vi "FctioTest.vi"(8 "error in":errorcluster, 9 "Invert Switch":bool, 10 "FPGA Reference In":refnum<k20>, 11 "DAQmx Task Name":refnum<k21>) -> (0 "error out":errorcluster, 2 "Individual Pin Result":bool[](array[boolean]), 3 "Test Pass":bool)   [LabVIEW 2018]
uses:
  Resources_Test/UART/ControlTestSlot.ctl
  <vilib>/DAQmx/read.llb/DAQmx Read (Digital 1D Bool NChan 1Samp 1Line).vi
  <vilib>/DAQmx/miscellaneous.llb/DAQmx Fill In Error Info.vi
panel:
  in  "Enum":T1
  in  "Resp Timeout":i32
  out "data":bool[](array[boolean])
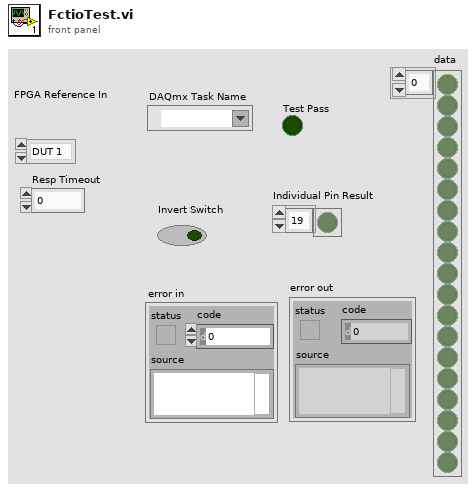
[diagram p1: front panel]
types:
  T1 = typedef "ControlTestSlot.ctl" = enum16{"DUT 1", "DUT 2"}
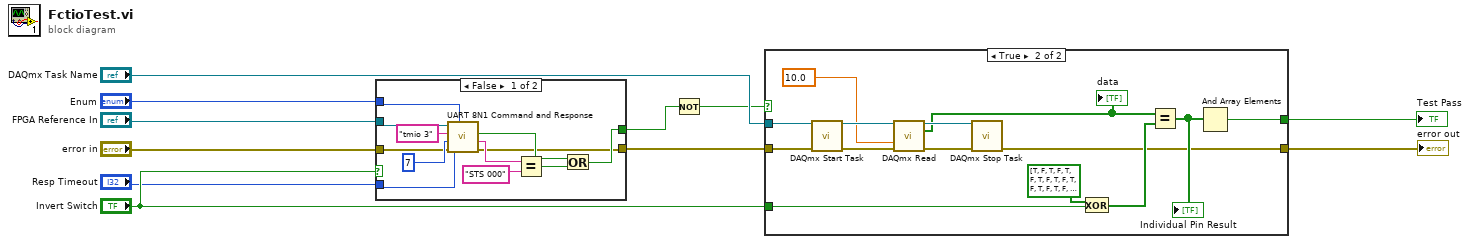
[diagram p0: block diagram]
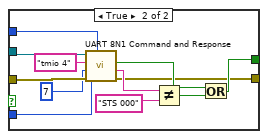
[diagram p3: hidden frame]
diagram:
  n1 = case shown="False" "Invert Switch" {
    tunnel: "error in" -> [w15 w35]
    tunnel: "FPGA Reference In" -> [w17 w34]
    tunnel: [w13 w24] -> w4
    tunnel: [w18 w26] -> w2
    tunnel: "Resp Timeout" -> [w14 w31]
    tunnel: "Enum" -> [w16 w32]
    frame False {
      n2 = call "UART 8N1 Command and Response.vi"("Response Timeout (ms)"=w14, "Enum"=w16, "Error In"=w15, "Response Size (char)"=u32 7, "Text to Send"="tmio 3", "FPGA Reference In"=w17) -> ("Error Out"=w13:errorcluster, "Received Text"=w22:string, "Timeout Flag"=w19:bool)  [unwired: 2 in, 1 out]
      n3 = Equal?(x=w22, y="STS 000") -> (x = y?=w20:bool)
      n4 = Or(x=w19, y=w20) -> (x .or. y?=w18:bool)
    }
    frame True {
      n5 = call "UART 8N1 Command and Response.vi"("Response Timeout (ms)"=w31, "Enum"=w32, "Error In"=w35, "Response Size (char)"=u32 7, "Text to Send"="tmio 4", "FPGA Reference In"=w34) -> ("Error Out"=w24:errorcluster, "Received Text"=w29:string, "Timeout Flag"=w25:bool)  [unwired: 2 in, 1 out]
      n6 = Not Equal?(x=w29, y="STS 000") -> (x != y?=w27:bool)
      n7 = Or(x=w25, y=w27) -> (x .or. y?=w26:bool)
    }
  }
  n8 = Not(x=w2) -> (.not. x?=w1:bool)
  n9 = case shown="True" w1 {
    selector: w1 -> [w37 _]
    tunnel: "DAQmx Task Name" -> [_ w51]
    tunnel: "Invert Switch" -> [_ w50]
    tunnel: [w36 w40] -> w5
    tunnel: w4 -> [w36 w39]
    tunnel: [w37 w38] -> w3
    frame False {
    }
    frame True {
      n10 = call <vilib>:"DAQmx Start Task.vi"("task/channels in"=w51, "error in"=w39) -> ("task out"=w48:refnum<k21>, "error out"=w49:errorcluster)  [unwired: 12 in]
      n11 = call-poly <vilib>:"DAQmx Read.vi"("task/channels in"=w48, "timeout"=10.0, "error in"=w49) -> ("task out"=w46:refnum<k21>, "data"=w42:bool[], "error out"=w45:errorcluster)  [unwired: 10 in]
      "data" <- w42
      n12 = call <vilib>:"DAQmx Stop Task.vi"("task/channels in"=w46, "error in"=w45) -> ("error out"=w40:errorcluster)  [unwired: 12 in, 1 out]
      n13 = Exclusive Or(1:w50, 2:bool[] [TRUE, FALSE, TRUE, FALSE, TRUE, FALSE, TRUE, FALSE, TRUE, FALSE, TRUE, FALSE, TRUE, FALSE, TRUE, FALSE, TRUE, FALSE] ("data")) -> (0:w44:bool[])
      n14 = Equal?(x=w42, y=w44) -> (x = y?=w43:bool[])
      "Individual Pin Result" <- w43
      n15 = And Array Elements(Boolean array=w43) -> (logical AND=w38:bool)
    }
  }
  "Test Pass" <- w3
  "error out" <- w5
